vi "main.vi"() -> ()   [LabVIEW 2016]
uses:
  Program Files (x86)/National Instruments/LabVIEW 2016/examples/Instrument IO/Serial/support/Serial - Settings.ctl
  2017-7-21/control1.ctl
  <vilib>/myRIO/Common/Instrument Driver Framework/myRIO v1.0/Encoder/typedefs/Encoder Signal Mode.ctl
  <vilib>/myRIO/Instrument Drivers/Onboard IO/DIO/typedefs/DIO Reference.ctl
  <vilib>/myRIO/Common/Instrument Driver Framework/Utilities/typedefs/myRIO Generic Hardware Reference.ctl
  <vilib>/myRIO/Common/Instrument Driver Framework/Utilities/typedefs/Hardware Version Enum.ctl
  <vilib>/myRIO/Common/Instrument Driver Framework/Utilities/typedefs/myRIO v1.0 Reference.ctl
  <vilib>/myRIO/Common/Instrument Driver Framework/Utilities/typedefs/Generic FPGA Reference.ctl
  <vilib>/myRIO/Common/Instrument Driver Framework/myRIO v1.0/DIO/typedefs/DIO Channels List.ctl
  <vilib>/myRIO/Common/Instrument Driver Framework/myRIO v1.0/DIO/typedefs/DIO Channels Enum.ctl
  <vilib>/userdefined/High Color/nirio_resource_hc.ctl
  <vilib>/myRIO/Common/Instrument Driver Framework/Utilities/vis/Is FPGA Ref Available.vi
  <vilib>/myRIO/Common/Instrument Driver Framework/myRIO v1.0/DIO/vis/myRIO v1.1 Open DIO.vi
  <vilib>/myRIO/Common/Instrument Driver Framework/Utilities/vis/Validate Channels.vi
  <vilib>/myRIO/Common/Instrument Driver Framework/myRIO v1.0/DIO/vis/myRIO v1.0 Reserve DIO.vi
  <vilib>/myRIO/Common/Instrument Driver Framework/myRIO v1.0/Resource Manager/vis/myRIO v1.0 Reserve Channel List.vi
  <vilib>/myRIO/Common/Instrument Driver Framework/myRIO v1.0/DIO/vis/myRIO v1.0 Build MUX Configuration DIO.vi
  <vilib>/myRIO/Common/Instrument Driver Framework/myRIO v1.0/Resource Manager/vis/myRIO v1.0 Reserve Channel.vi
  <vilib>/myRIO/Common/Instrument Driver Framework/myRIO v1.0/Resource Manager/vis/myRIO v1.0 Unreserve Channel.vi
  <vilib>/myRIO/Common/Instrument Driver Framework/myRIO v1.0/Resource Manager/vis/myRIO v1.0 Create Configuration List.vi
  <vilib>/myRIO/Common/Instrument Driver Framework/myRIO v1.0/Resource Manager/vis/myRIO v1.0 Build Mutex Name.vi
  <vilib>/Instr/_visa.llb/VISA Configure Serial Port (Instr).vi
  <vilib>/Utility/error.llb/Error Cluster From Error Code.vi
  <vilib>/myRIO/Common/Instrument Driver Framework/myRIO v1.0/DIO/vis/myRIO v1.0 Write DIO.vi
  <vilib>/myRIO/Common/Instrument Driver Framework/myRIO v1.0/Encoder/vis/myRIO v1.0 Read Encoder.vi
  <vilib>/Utility/VariantDataType/GetNumericInfo.vi
  <vilib>/myRIO/Common/Instrument Driver Framework/myRIO v1.0/myRIO v1.1 Open.vi
  <vilib>/myRIO/Common/Instrument Driver Framework/Utilities/vis/IO Manager.vi
  <vilib>/myRIO/Common/Instrument Driver Framework/Utilities/vis/Configuration Manager.vi
  <vilib>/myRIO/Common/Instrument Driver Framework/myRIO v1.0/Resource Manager/vis/myRIO v1.0 Configure IO.vi
  <vilib>/myRIO/Common/Instrument Driver Framework/myRIO v1.0/myRIO v1.0 Close.vi
  <vilib>/myRIO/Express VI/Onboard IO/DO/DO Express VI.xnode
  <vilib>/myRIO/Instrument Drivers/Onboard IO/DIO/vis/myRIO DIO Open.xnode
  <vilib>/myRIO/Instrument Drivers/Onboard IO/DIO/DIO.lvlib
  <vilib>/myRIO/Instrument Drivers/Onboard IO/Encoder/Encoder.lvlib
panel:
  out "调整的角度1":dbl
  out "长度":i32
  out "4（找球、捡球）":bool
  out "3（移动）":bool
  out "2（投球）":bool
  out "1（捡球）":bool
  out "0（无命令）":bool
  out "收到X坐标":i32
  out "收到Y坐标":i32
  out "收到的角度":dbl
  out "收到的状态":i32
  out "x轴":dbl
  out "Y轴":dbl
  out "Counter Value":i32
  out "x*y":dbl
  out "read buffer":string
  out "读取缓冲区":string
  in  "停止":bool
  in  "写入":bool
  out "角度":dbl
  out "角度 弧度":dbl
  in  "调整":dbl
  out "调整后 角度值":dbl
  in  "A/DIO0 (Pin 11)":bool
  out "建立通信":errorcluster caption="错误输出"
  out "收到的数据":string
  out "发送":string
  out "发送的标志位":string="0"
  out "发送的角度":string
  out "Y轴字符串":string
  out "X轴字符串":string
  # "东南大学篮球机器机器人下位机"
  # "室内定位"
  # "通信"
  # "数据解析"
  # "电子罗盘"
  # "脚轮"
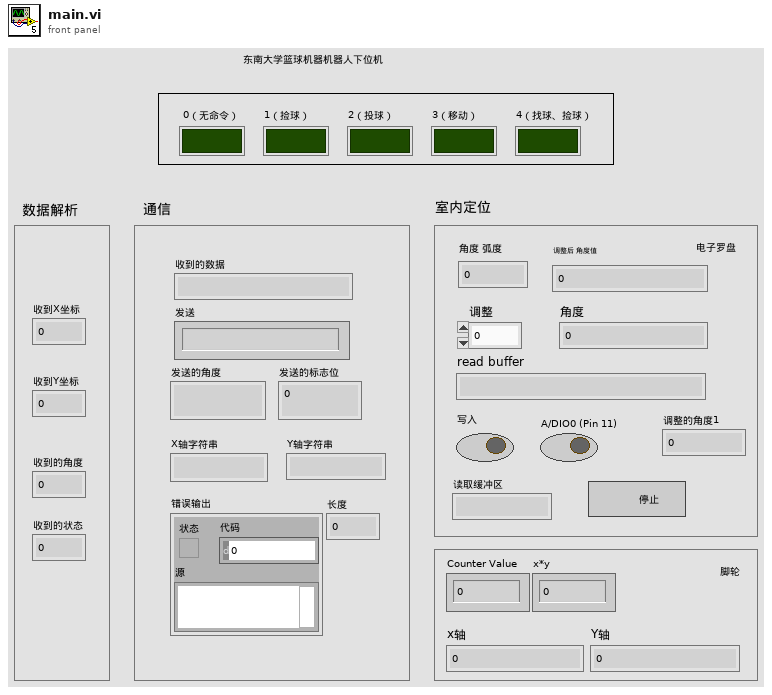
[diagram p1: front panel]
types:
  T1 = typedef "control1.ctl" = cluster{"XON":enum16{"NUL", "SOH", "STX", "ETX", "EOT", "ENQ", "ACK", "BEL", "BS", "HT", "LF", "VT", "FF", "CR", "SO", "SI", "DLE", "DC1", "DC2", "DC3", "DC4", "NAK", "SYN", "ETB", "CAN", "EM", "SUB", "ESC", "FS", "GS", "RS", "US", "SP", "!", "\"", "#", "$", "%", "&", "'", "(", ")", "*", "+", ",", "- (-)", ".", "/", "0", "1", "2", "3", "4", "5", "6", "7", "8", "9", ":", ";", "<", "=", ">", "?", "@", "A", "B", "C", "D", "E", "F", "G", "H", "I", "J", "K", "L", "M", "N", "O", "P", "Q", "R", "S", "T", "U", "V", "W", "X", "Y", "Z", "[", "\\", "]", "^", "_", "`", "a", "b", "c", "d", "e", "f", "g", "h", "i", "j", "k", "l", "m", "n", "o", "p", "q", "r", "s", "t", "u", "v", "w", "x", "y", "z", "{", "|", "}", "~"}, "XOFF":enum16{"NUL", "SOH", "STX", "ETX", "EOT", "ENQ", "ACK", "BEL", "BS", "HT", "LF", "VT", "FF", "CR", "SO", "SI", "DLE", "DC1", "DC2", "DC3", "DC4", "NAK", "SYN", "ETB", "CAN", "EM", "SUB", "ESC", "FS", "GS", "RS", "US", "SP", "!", "\"", "#", "$", "%", "&", "'", "(", ")", "*", "+", ",", "- (-)", ".", "/", "0", "1", "2", "3", "4", "5", "6", "7", "8", "9", ":", ";", "<", "=", ">", "?", "@", "A", "B", "C", "D", "E", "F", "G", "H", "I", "J", "K", "L", "M", "N", "O", "P", "Q", "R", "S", "T", "U", "V", "W", "X", "Y", "Z", "[", "\\", "]", "^", "_", "`", "a", "b", "c", "d", "e", "f", "g", "h", "i", "j", "k", "l", "m", "n", "o", "p", "q", "r", "s", "t", "u", "v", "w", "x", "y", "z", "{", "|", "}", "~"}}
  T2 = typedef "Serial - Settings.ctl" = cluster{"波特率":u32, "数据位":u16, "校验":enum16{"None", "Odd", "Even", "Mark", "Space"}, "停止位":u16, "流控制":u16}
  T3 = typedef "DIO.lvlib/DIO Reference.ctl" = cluster{"myRIO Reference":T4, "DIO Channels List":T8}
  T4 = typedef "myRIO Generic Hardware Reference.ctl" = cluster{"myRIO Model":T5, "myRIO Hardware Reference":T6}
  T5 = typedef "Hardware Version Enum.ctl" = enum16{"Unknown", "myRIO-1900", "myRIO-1950", "roboRIO", "NI ELVIS RIO CM"}
  T6 = typedef "myRIO v1.0 Reference.ctl" = cluster{"Generic FPGA Reference":T7, "Allow multiple opens":bool}
  T7 = typedef "Generic FPGA Reference.ctl" = refnum<k20>
  T8 = typedef "DIO Channels List.ctl" = T9[]
  T9 = typedef "DIO Channels Enum.ctl" = enum16{"Not Connected", "C/DIO0", "C/DIO1", "C/DIO2", "C/DIO3", "C/DIO4", "C/DIO5", "C/DIO6", "C/DIO7", "A/DIO0", "A/DIO1", "A/DIO2", "A/DIO3", "A/DIO4", "A/DIO5", "A/DIO6", "A/DIO7", "A/DIO8", "A/DIO9", "A/DIO10", "A/DIO11", "A/DIO12", "A/DIO13", "A/DIO14", "A/DIO15", "B/DIO0", "B/DIO1", "B/DIO2", "B/DIO3", "B/DIO4", "B/DIO5", "B/DIO6", "B/DIO7", "B/DIO8", "B/DIO9", "B/DIO10", "B/DIO11", "B/DIO12", "B/DIO13", "B/DIO14", "B/DIO15", "LED0", "LED1", "LED2", "LED3", "Button0", "DIO/DIO0", "DIO/DIO1", "DIO/DIO2", "DIO/DIO3", "DIO/DIO4", "DIO/DIO5", "DIO/DIO6", "DIO/DIO7", "DIO/DIO8", "DIO/DIO9", "SPI/CS0", "SPI/CS1", "SPI/CS2", "SPI/CS3", "LED RADIO (Green)", "LED RADIO (Red)", "LED COMM (Green)", "LED COMM (Red)", "LED MODE (Green)", "LED MODE (Red)"}
  T10 = typedef "nirio_resource_hc.ctl" = tag
  T11 = typedef "Encoder Signal Mode.ctl" = enum16{"Quadrature phase signal", "Step and direction signal"}
  T12 = typedef "PWM.lvlib/PWM Reference.ctl" = cluster{"myRIO Reference":T4, "PWM Channels Enum":T13, "PWM Configuration":T14}
  T13 = typedef "PWM Channels Enum.ctl" = enum16{"Not Connected", "C/PWM0", "C/PWM1", "A/PWM0", "A/PWM1", "A/PWM2", "B/PWM0", "B/PWM1", "B/PWM2", "PWM/PWM0", "PWM/PWM1", "PWM/PWM2", "PWM/PWM3", "PWM/PWM4", "PWM/PWM5", "PWM/PWM6", "PWM/PWM7", "PWM/PWM8", "PWM/PWM9"}
  T14 = typedef "PWM.lvlib/PWM Configuration.ctl" = cluster{"Frequency":dbl, "Duty Cycle":dbl}
  T15 = enum16{"NUL", "SOH", "STX", "ETX", "EOT", "ENQ", "ACK", "BEL", "BS", "HT", "LF", "VT", "FF", "CR", "SO", "SI", "DLE", "DC1", "DC2", "DC3", "DC4", "NAK", "SYN", "ETB", "CAN", "EM", "SUB", "ESC", "FS", "GS", "RS", "US", "SP", "!", "\"", "#", "$", "%", "&", "'", "(", ")", "*", "+", ",", "- (-)", ".", "/", "0", "1", "2", "3", "4", "5", "6", "7", "8", "9", ":", ";", "<", "=", ">", "?", "@", "A", "B", "C", "D", "E", "F", "G", "H", "I", "J", "K", "L", "M", "N", "O", "P", "Q", "R", "S", "T", "U", "V", "W", "X", "Y", "Z", "[", "\\", "]", "^", "_", "`", "a", "b", "c", "d", "e", "f", "g", "h", "i", "j", "k", "l", "m", "n", "o", "p", "q", "r", "s", "t", "u", "v", "w", "x", "y", "z", "{", "|", "}", "~"}
  T16 = typedef "Encoder.lvlib/Encoder Reference.ctl" = cluster{"myRIO Reference":T4, "Encoder Channels Enum":T17}
  T17 = typedef "Encoder Channels Enum.ctl" = enum16{"Not Connected", "C/ENC0", "C/ENC1", "A/ENC", "B/ENC", "DIO/ENC0", "DIO/ENC1", "DIO/ENC2", "DIO/ENC3", "DIO/ENC4"}
  T18 = cluster{"PWM Ref Out":T12, "PWM Ref Out":T12, "PWM Ref Out":T12, "PWM Ref Out":T12, "DIO Ref Out":T3}
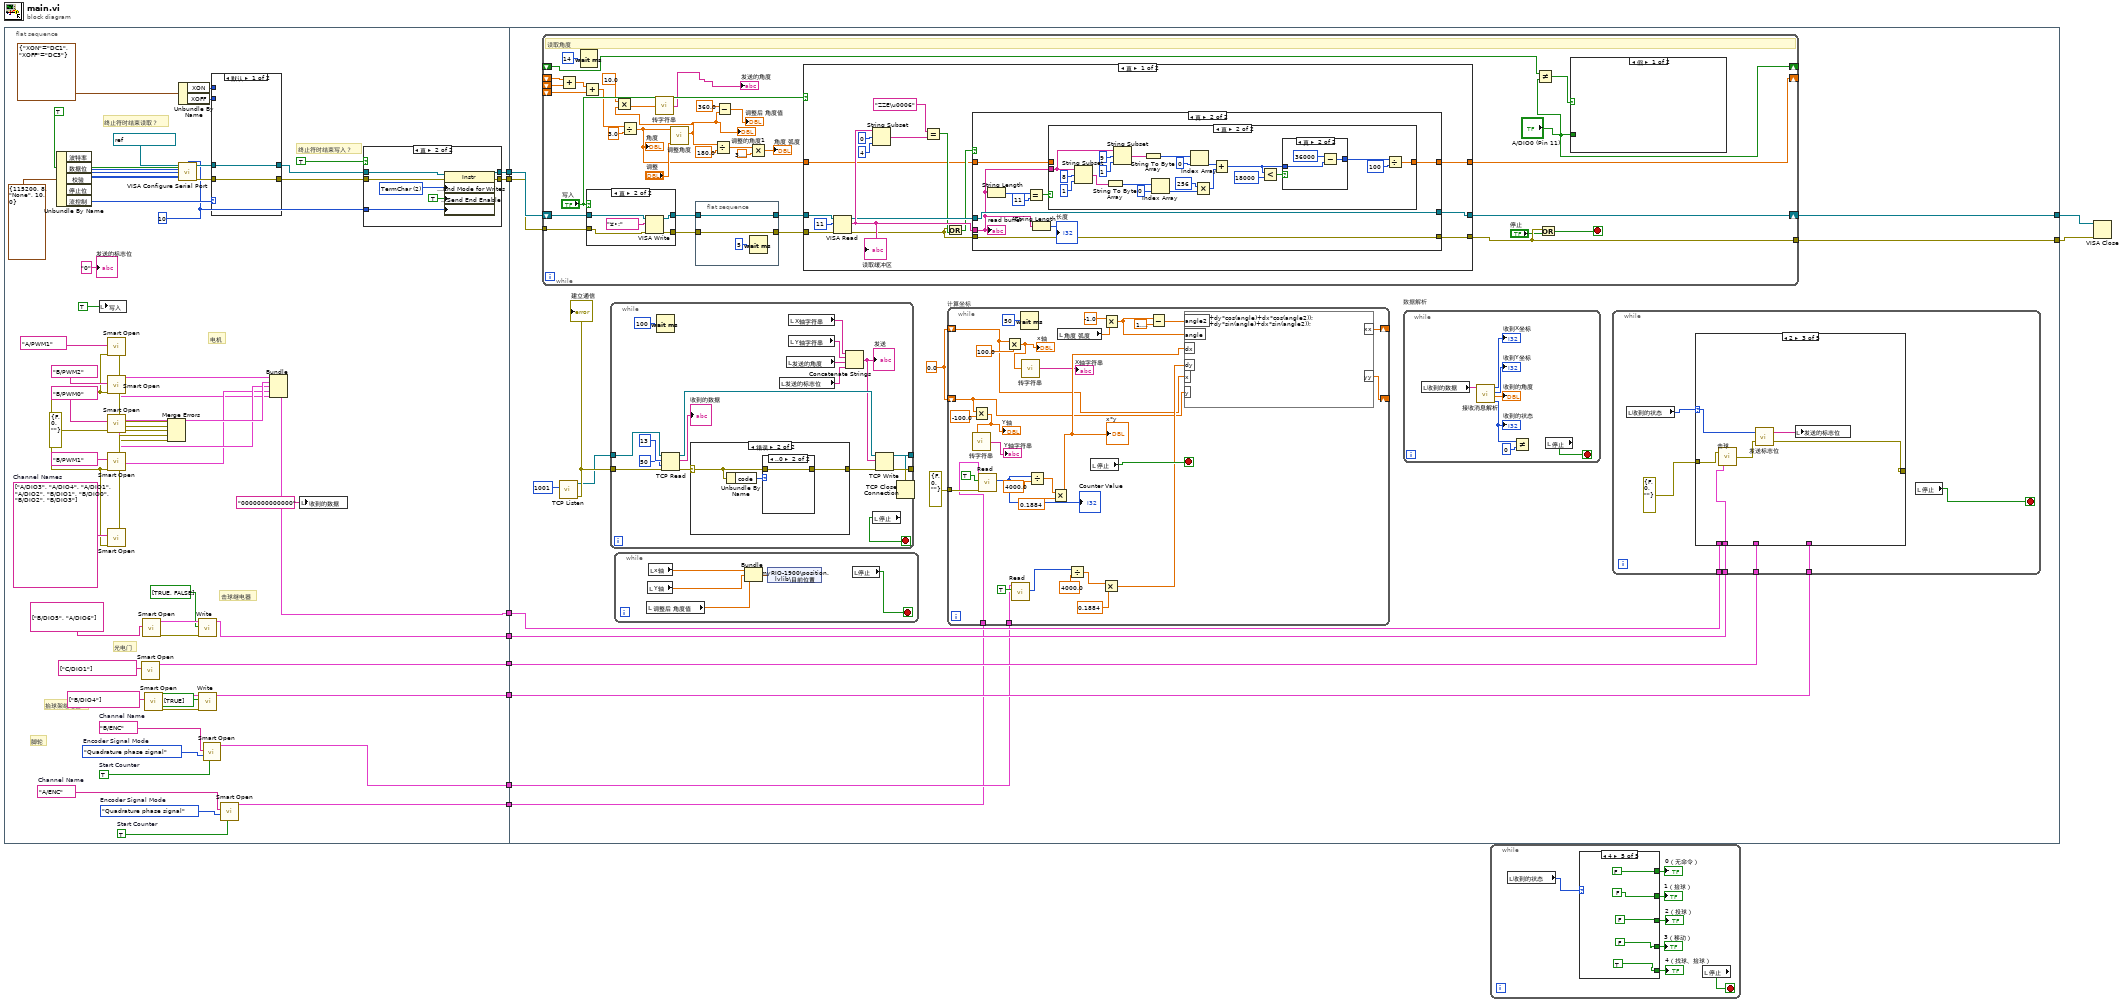
[diagram p0: block diagram]
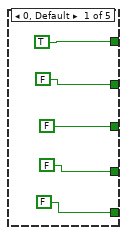
[diagram p2: hidden frame]
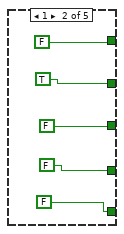
[diagram p3: hidden frame]
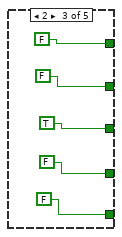
[diagram p4: hidden frame]
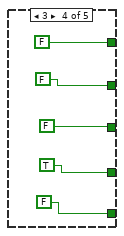
[diagram p5: hidden frame]
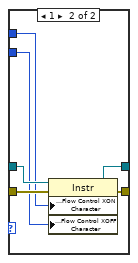
[diagram p7: hidden frame]
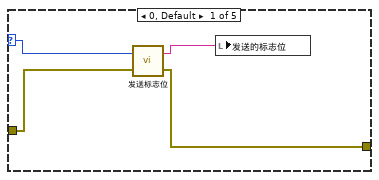
[diagram p8: hidden frame]
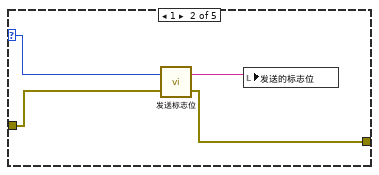
[diagram p9: hidden frame]
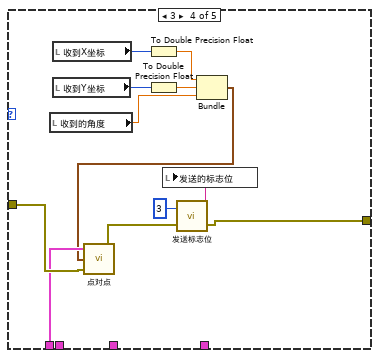
[diagram p10: hidden frame]
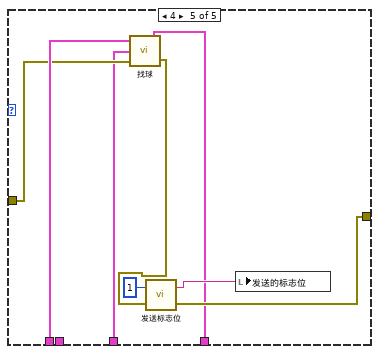
[diagram p11: hidden frame]
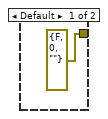
[diagram p13: hidden frame]
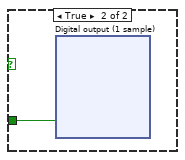
[diagram p14: hidden frame]
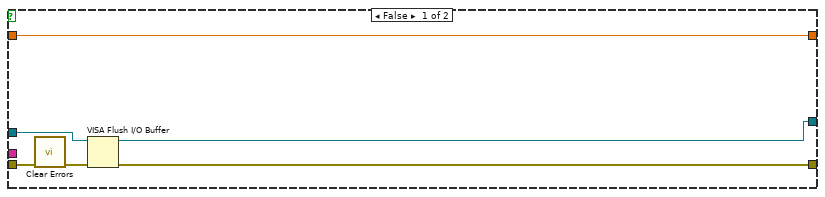
[diagram p16: hidden frame]
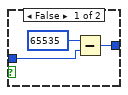
[diagram p18: hidden frame]
diagram:
  n1 = flat-sequence {
    tunnel: [w34] -> w10
    tunnel: [w33] -> w9
    tunnel: [w32] -> w6
    tunnel: [w26] -> w5
    tunnel: [w24] -> w4
    tunnel: [w19] -> w3
    tunnel: [w15] -> w2
    tunnel: [w11] -> w1
    tunnel: w10 -> [w103]
    tunnel: w9 -> [w102]
    tunnel: [w101] -> w8
    tunnel: [w100] -> w7
    tunnel: w6 -> [w92]
    tunnel: w5 -> [w91]
    tunnel: w4 -> [w90]
    tunnel: w3 -> [w89]
    tunnel: w2 -> [w88]
    tunnel: w1 -> [w87]
    frame #0 {
      w12 = TRUE  # Start Counter
      w13 = Encoder_Signal_Mode."Quadrature phase signal"  # Encoder Signal Mode
      w14 = tag "A/ENC"  # Channel Name
      w16 = TRUE  # Start Counter
      w17 = Encoder_Signal_Mode."Quadrature phase signal"  # Encoder Signal Mode
      w18 = tag "B/ENC"  # Channel Name
      w62 = errorcluster {"status"=FALSE, "code"=0, "source"=""} ("错误输入")
      w37 = u8 10 ("终止符")
      w63 = tag[] ["A/DIO3", "A/DIO4", "A/DIO1", "A/DIO2", "B/DIO1", "B/DIO0", "B/DIO2", "B/DIO3"]  # Channel Names
      # "脚轮"
      # "抬球架继电器"
      # "光电门"
      # "电机"
      # "击球继电器"
      # "终止符时结束读取？"
      # "终止符时结束写入？"
      n2 = Unbundle By Name(T2 {"波特率"=115200, "数据位"=8, "校验"=enum."None", "停止位"=10, "流控制"=0} ("串口设置")) -> ("波特率"=w44:u32, "数据位"=w45:u16, "校验"=w46:enum16{"None", "Odd", "Even", "Mark", "Space"}, "停止位"=w47:u16, "流控制"=w42:u16)
      n3 = local write "写入"(TRUE ("写入")) -> ()
      n4 = call <vilib>:"Smart Open.vi"("error in (no error)"=w62, "Channel Name"=tag "A/PWM1") -> ("error out"=w61:errorcluster, "PWM Ref Out"=w56:T12)  [unwired: 8 in]
      n5 = call <vilib>:"Smart Open.vi"("error in (no error)"=w62, "Channel Name"=tag "B/PWM2") -> ("error out"=w60:errorcluster, "PWM Ref Out"=w55:T12)  [unwired: 8 in]
      n6 = call <vilib>:"Smart Open.vi"("error in (no error)"=w62, "Channel Name"=tag "B/PWM0") -> ("error out"=w59:errorcluster, "PWM Ref Out"=w54:T12)  [unwired: 8 in]
      n7 = call <vilib>:"Smart Open.vi"("error in (no error)"=w62, "Channel Name"=tag "B/PWM1") -> ("error out"=w58:errorcluster, "PWM Ref Out"=w53:T12)  [unwired: 8 in]
      n8 = call <vilib>:"Smart Open.vi"("error in (no error)"=w62, "Channel Names"=w63) -> ("error out"=w57:errorcluster, "DIO Ref Out"=w52:T3)  [unwired: 8 in]
      n9 = call <vilib>:"Smart Open.vi"("Channel Names"=tag[] ["C/DIO1"]) -> ("DIO Ref Out"=w24:T3)  [unwired: 9 in, 1 out]
      n10 = call <vilib>:"Smart Open.vi"("Channel Names"=tag[] ["B/DIO5", "A/DIO6"]) -> ("error out"=w27:errorcluster, "DIO Ref Out"=w29:T3)  [unwired: 9 in]
      n11 = call <vilib>:"Smart Open.vi"("Channel Names"=tag[] ["B/DIO4"]) -> ("error out"=w21:errorcluster, "DIO Ref Out"=w22:T3)  [unwired: 9 in]
      n12 = Merge Errors(w61, w60, w59, w58, w57) -> ()  [unwired: 1 out]
      n13 = Unbundle By Name(T1 {"XON"=enum."DC1", "XOFF"=enum."DC3"}) -> ("XON"=w41:T15, "XOFF"=w40:T15)
      n14 = call-poly "VISA Configure Serial Port"("VISA resource name"=refnum<visa-resource-name> "ASRL2::INSTR" ("VISA资源名称"), "termination char\n(0xA = '\\n' = LF)"=w37, "Enable Termination\nChar (T)"=TRUE, "baud rate (9600)"=w44, "data bits (8)"=w45, "parity (0:none)"=w46, "stop bits (10: 1 bit)"=w47, "flow control (0:none)"=w42) -> ("VISA resource name out"=w48:refnum<visa-resource-name>, "error out"=w49:errorcluster)  [unwired: 2 in, 4 out]
      n15 = call <vilib>:"Write.vi"("error in (no error)"=w27, "Values"=bool[] [TRUE, FALSE], "DIO Ref In"=w29) -> ("DIO Ref Out"=w26:T3)  [unwired: 6 in, 1 out]
      n16 = call <vilib>:"Write.vi"("error in (no error)"=w21, "Values"=bool[] [TRUE], "DIO Ref In"=w22) -> ("DIO Ref Out"=w19:T3)  [unwired: 6 in, 1 out]
      n17 = call <vilib>:"Smart Open.vi"("Start Counter"=w16, "Encoder Signal Mode"=w17, "Channel Name"=w18) -> ("Encoder Ref Out"=w15:T16)  [unwired: 7 in, 1 out]
      n18 = case shown="默认" w42 {
        tunnel: [w79 w86] -> w39
        tunnel: [w80 w85] -> w38
        tunnel: w49 -> [w79 w84]
        tunnel: w48 -> [w80 w83]
        tunnel: w41 -> [_ w82]
        tunnel: w40 -> [_ w81]
        frame Default {
        }
        frame 1 {
          n19 = property class="Instr"(reference=w83, error in=w84, "Serial Settings:Flow Control XON Character"=w82, "Serial Settings:Flow Control XOFF Character"=w81) -> (reference out=w85:refnum<visa-resource-name>, error out=w86:errorcluster)
        }
      }
      n20 = call <vilib>:"Smart Open.vi"("Start Counter"=w12, "Encoder Signal Mode"=w13, "Channel Name"=w14) -> ("Encoder Ref Out"=w11:T16)  [unwired: 7 in, 1 out]
      n21 = Bundle("PWM Ref Out"=w56, "PWM Ref Out"=w55, "PWM Ref Out"=w54, "PWM Ref Out"=w53, "DIO Ref Out"=w52) -> (w32:T18)  [unwired: 1 in]
      n22 = local write "收到的数据"("0000000000000" ("收到的数据")) -> ()
      n23 = case shown="真" TRUE {
        tunnel: w38 -> [w70 w78]
        tunnel: w39 -> [w71 w77]
        tunnel: [w70 w76] -> w34
        tunnel: [w71 w75] -> w33
        tunnel: w37 -> [_ w73]
        frame False {
        }
        frame True {
          w74 = u16 2 items=["None", "LastBit", "TermChar", "Break"] ("Serial Settings:Serial End Mode for Writes")
          n24 = property class="Instr"(reference=w78, error in=w77, "Serial Settings:End Mode for Writes"=w74, "Message Based Settings:Send End Enable"=TRUE, "Message Based Settings:Termination Character"=w73) -> (reference out=w76:refnum<visa-resource-name>, error out=w75:errorcluster)
        }
      }
      "发送的标志位" <- "0" ("发送的标志位")
    }
    frame #1 {
      w94 = 0.0
      n25 = while {
        shift-right: [w245] -> w100
        shift-left: w103 -> [w244]
        tunnel: [w242] -> w101
        shift-right: [w234] -> _
        shift-left: _ -> [w233]
        shift-left: _ -> [w232]
        shift-left: _ -> [w230]
        shift-right: ["A/DIO0 (Pin 11)"] -> _
        shift-left: _ -> [w220]
        tunnel: w102 -> [w219]
        stop <- w243 stop-if-true
        # "读取角度"
        n26 = Add(x=w233, y=w232) -> (x+y=w231:dbl)
        n27 = Wait (ms)(milliseconds to wait=u32 14) -> ()  [unwired: 1 out]
        n28 = Add(x=w231, y=w230) -> (x+y=w229:dbl)
        n29 = case shown="真" "写入" {
          tunnel: w244 -> [w286 w290]
          tunnel: [w286 w289] -> w240
          tunnel: [w285 w288] -> w239
          tunnel: w219 -> [w285 w287]
          frame False {
          }
          frame True {
            n30 = VISA Write(VISA resource name=w290, write buffer="¥•:" ("命令"), error in (no error)=w287) -> (VISA resource name out=w289:refnum<visa-resource-name>, error out=w288:errorcluster)  [unwired: 1 out]
          }
        }
        n31 = Divide(x=w229, y=3.0) -> (x/y=w215:dbl)
        "角度" <- w215
        n32 = call "调整角度.vi"("调整"="调整", "原角度"=w215) -> ("调整后 角度值"=w212:dbl)  [unwired: 9 in]
        "调整的角度1" <- w212
        n33 = Multiply(x=10.0, y=w212) -> (x*y=w217:dbl)
        n34 = call "转字符串.vi"("输入"=w217) -> ("结果字符串"=→"发送的角度":string)
        n35 = flat-sequence {
          tunnel: w240 -> [w283]
          tunnel: w239 -> [w284]
          tunnel: [w284] -> w238
          tunnel: [w283] -> w237
          frame #0 {
            n36 = Wait (ms)(milliseconds to wait=u32 5) -> ()  [unwired: 1 out]
          }
        }
        n37 = Divide(x=w212, y=180.0) -> (x/y=w225:dbl)
        n38 = Subtract(x=360.0, y=w212) -> (x-y=→"调整后 角度值":dbl)
        n39 = Multiply(x=w225, y=3.141592653589793) -> (x*y=→"角度 弧度":dbl)
        n40 = case shown="真" "写入" {
          tunnel: [w300 w352] -> w245
          tunnel: [w294 w353] -> w242
          tunnel: w238 -> [w299 w353]
          tunnel: w237 -> [w298 w352]
          tunnel: [w293 w351] -> w234
          tunnel: w215 -> [w292 w351]
          frame True {
            n41 = VISA Read(VISA resource name=w298, byte count=u32 11 ("读数"), error in (no error)=w299) -> (VISA resource name out=w301:refnum<visa-resource-name>, read buffer=w302:string, error out=w295:errorcluster)  [unwired: 1 out]
            "读取缓冲区" <- w302
            n42 = String Subset(string=w302, offset (0)=0 ("偏移量(0)"), length (rest)=4 ("长度（剩余）")) -> (substring=w304:string)
            n43 = Equal?(x="ZZE\u0006", y=w304) -> (x = y?=w297:bool)
            n44 = Or(x=w295, y=w297) -> (x .or. y?=w296:bool)
            n45 = case shown="真" w296 {
              tunnel: w302 -> [_ w315]
              tunnel: w301 -> [w313 w322]
              tunnel: [w312 w322] -> w300
              tunnel: w295 -> [w311 w321]
              tunnel: [w309 w321] -> w294
              tunnel: [w308 w317] -> w293
              tunnel: w292 -> [w308 w316]
              frame False {
                n46 = call <vilib>:"Clear Errors.vi"("error in (no error)"=w311) -> ("error out"=w310:errorcluster)  [unwired: 5 in, 1 out]
                n47 = VISA Flush I/O Buffer(VISA resource name=w313, error in (no error)=w310) -> (VISA resource name out=w312:refnum<visa-resource-name>, error out=w309:errorcluster)  [unwired: 1 in]
              }
              frame True {
                n48 = String Length(string=w315) -> (length=w318:i32)
                n49 = Equal?(x=w318, y=11) -> (x = y?=w320:bool)
                n50 = String Length(string=w315) -> (length=→"长度":i32)
                n51 = case shown="真" w320 {
                  tunnel: w315 -> [_ w332]
                  tunnel: [w323 w324] -> w317
                  tunnel: w316 -> [w323 _]
                  frame False {
                  }
                  frame True {
                    n52 = String Subset(string=w332, offset (0)=8 ("偏移量(0)"), length (rest)=1 ("长度（剩余）")) -> (substring=w342:string)
                    n53 = String To Byte Array(string=w342) -> (unsigned byte array=w341:u8[])
                    n54 = String Subset(string=w332, offset (0)=9 ("偏移量(0)"), length (rest)=1 ("长度（剩余）")) -> (substring=w335:string)
                    n55 = String To Byte Array(string=w335) -> (unsigned byte array=w336:u8[])
                    n56 = Index Array(array=w341, index=0 ("索引")) -> (element=w339:u8)
                    n57 = Index Array(array=w336, index=0 ("索引")) -> (element=w331:u8)
                    n58 = Multiply(x=256, y=w339) -> (x*y=w330:i32)
                    n59 = Add(x=w331, y=w330) -> (x+y=w327:i32)
                    n60 = Less?(x=w327, y=18000) -> (x < y?=w328:bool)
                    n61 = case shown="真" w328 {
                      tunnel: w327 -> [w345 w350]
                      tunnel: [w347 w348] -> w326
                      frame False {
                        n62 = Subtract(x=65535 ("y"), y=w345) -> (x-y=w347:i32)
                      }
                      frame True {
                        n63 = Subtract(x=36000, y=w350) -> (x-y=w348:i32)
                      }
                    }
                    n64 = Divide(x=w326, y=100) -> (x/y=w324:dbl)
                  }
                }
                "read buffer" <- w315
              }
            }
          }
          frame False {
          }
        }
        n65 = Not Equal?(x=w220, y="A/DIO0 (Pin 11)") -> (x != y?=w222:bool)
        n66 = Or(x=w242, y="停止") -> (x .or. y?=w243:bool)
        n67 = case shown="假" w222 {
          tunnel: "A/DIO0 (Pin 11)" -> [_ w246]
          frame False {
          }
          frame True {
            n68 = xnode "Digital output (1 sample)"("A/DIO1 (Pin 13)"=w246) -> ()  [unwired: 1 in, 1 out]
          }
        }
      }
      n69 = call <vilib>:"TCP Listen.vi"("port"=u16 1001 ("远程端口或服务名称")) -> ("error out"=w99:errorcluster, "connection ID"=w95:refnum<k5>)  [unwired: 6 in, 3 out]
      "建立通信" <- w99
      n70 = while {
        tunnel: w95 -> [w205]
        tunnel: w99 -> [w204]
        tunnel: [w199] -> w96
        tunnel: [w197] -> w97
        stop <- w189 stop-if-true
        n71 = Wait (ms)(milliseconds to wait=100) -> ()  [unwired: 1 out]
        n72 = TCP Read(connection ID=w205, bytes to read=13 ("读取的字节"), error in (no error)=w204, 9:50) -> (connection ID out=w200:refnum<k5>, data out=→"收到的数据":string, error out=w202:errorcluster)  [unwired: 1 in]
        n73 = case shown="错误" w202 {
          selector: w202 -> [w206 w207]
          tunnel: [w206 w208] -> w198
          frame No Error {
          }
          frame Error {
            n74 = Unbundle By Name(w207) -> ("code"=w209:i32)
            n75 = case shown="..0" w209 {
              tunnel: [errorcluster {"status"=FALSE, "code"=0, "source"=""} ("error IO") w211] -> w208
              tunnel: w207 -> [_ w211]
              frame Default {
              }
              frame ..0 {
              }
            }
          }
        }
        n76 = local read "发送的标志位"() -> (w191:string)
        n77 = local read "发送的角度"() -> (w190:string)
        n78 = local read "X轴字符串"() -> (w194:string)
        n79 = local read "Y轴字符串"() -> (w193:string)
        n80 = Concatenate Strings(w194, w193, w190, w191) -> (w192:string)
        "发送" <- w192
        n81 = local read "停止"() -> (w189:bool)
        n82 = TCP Write(connection ID=w200, data in=w192, error in (no error)=w198) -> (connection ID out=w199:refnum<k5>, error out=w197:errorcluster)  [unwired: 1 in, 1 out]
      }
      n83 = while {
        stop <- w104 stop-if-true
        n84 = local read "调整后 角度值"() -> (w106:dbl)
        n85 = local read "Y轴"() -> (w107:dbl)
        n86 = local read "x轴"() -> (w108:dbl)
        n87 = Bundle("x轴"=w108, "Y轴"=w107, "调整后 角度值"=w106) -> (w105:cluster{"x轴":dbl, "Y轴":dbl, "调整后 角度值":dbl})  [unwired: 1 in]
        n88 = shared-variable "myRIO-1900\\position.lvlib\\目前位置"(w105) -> ()  [unwired: 1 in, 1 out]
        n89 = local read "停止"() -> (w104:bool)
      }
      n90 = TCP Close Connection(connection ID=w96, error in (no error)=w97) -> ()  [unwired: 1 in, 2 out]
      n91 = while "计算坐标" {
        shift-right: [w187] -> _
        shift-left: w94 -> [w171]
        shift-right: [w186] -> _
        shift-left: w94 -> [w172]
        tunnel: errorcluster {"status"=FALSE, "code"=0, "source"=""} ("错误常量") -> [w161]
        tunnel: w88 -> [w163]
        tunnel: w87 -> [w159]
        stop <- w188 stop-if-true
        n92 = Multiply(x=w172, y=-100.0) -> (x*y=w158:dbl)
        "Y轴" <- w158
        n93 = call "转字符串.vi"("输入"=w158) -> ("结果字符串"=→"Y轴字符串":string)
        n94 = call <vilib>:"Read.vi"("error in (no error)"=w161, "Reset Counter"=TRUE, "Encoder Ref In"=w159) -> ("Counter Value"=w162:i32)  [unwired: 4 in, 4 out]
        "Counter Value" <- w162
        n95 = Multiply(x=w171, y=100.0) -> (x*y=w157:dbl)
        "x轴" <- w157
        n96 = call <vilib>:"Read.vi"("Reset Counter"=TRUE, "Encoder Ref In"=w163) -> ("Counter Value"=w164:i32)  [unwired: 5 in, 4 out]
        n97 = Wait (ms)(milliseconds to wait=u32 50 ("等待时间（毫秒）")) -> ()  [unwired: 1 out]
        n98 = call "转字符串.vi"("输入"=w157) -> ("结果字符串"=→"X轴字符串":string)
        n99 = Divide(x=w162, y=4000.0) -> (x/y=w182:dbl)
        n100 = Multiply(x=w182, y=0.1884) -> (x*y=w180:dbl)
        "x*y" <- w180
        n101 = local read "角度 弧度"() -> (w170:dbl)
        n102 = Divide(x=w164, y=4000.0) -> (x/y=w178:dbl)
        n103 = local read "停止"() -> (w188:bool)
        n104 = Multiply(x=w178, y=0.1884) -> (x*y=w176:dbl)
        n105 = Multiply(x=-1.0, y=w170) -> (x*y=w168:dbl)
        n106 = Subtract(x=w168, y=1.5707963267948966) -> (x-y=w185:dbl)
        n107 = formula code="xx=(x+dy*cos(angle)+dx*cos(angle2));\nyy=(y+dy*sin(angle)+dx*sin(angle2));"("angle"=w168, "dx"=w180, "dy"=w176, "x"=w171, "y"=w172, "angle2"=w185) -> ("xx"=w187:dbl, "yy"=w186:dbl)
      }
      n108 = while "数据解析" {
        stop <- w156 stop-if-true
        n109 = local read "收到的数据"() -> (w150:string)
        n110 = call "接收消息解析.vi"("上位机消息"=w150) -> ("状态"=w155:i32, "角度"=→"收到的角度":dbl, "Y"=→"收到Y坐标":i32, "X"=→"收到X坐标":i32)  [unwired: 7 in]
        "收到的状态" <- w155
        n111 = Not Equal?(x=w155, y=0) -> ()  [unwired: 1 out]
        n112 = local read "停止"() -> (w156:bool)
      }
      n113 = while {
        tunnel: w92 -> [w112]
        tunnel: w91 -> [w111]
        tunnel: w90 -> [w110]
        tunnel: w89 -> [w109]
        stop <- w115 stop-if-true
        n114 = local read "收到的状态"() -> (w113:i32)
        n115 = case shown="2" w113 {
          selector: w113 -> [w119 w123 w127 _ _]
          tunnel: errorcluster {"status"=FALSE, "code"=0, "source"=""} ("error out") -> [w117 w121 w125 w139 w144]
          tunnel: [w116 w120 w128 w130 w148] -> _
          tunnel: w112 -> [_ _ _ w137 w145]
          tunnel: w111 -> [_ _ w124 _ _]
          tunnel: w110 -> [_ _ _ _ w143]
          tunnel: w109 -> [_ _ _ _ w142]
          frame 0, Default {
            n116 = call "发送标志位.vi"("error out 2"=w117, "数值"=w119) -> ("error out"=w116:errorcluster, "十进制整型字符串"=w118:string)
            n117 = local write "发送的标志位"(w118) -> ()
          }
          frame 1 {
            n118 = call "发送标志位.vi"("error out 2"=w121, "数值"=w123) -> ("error out"=w120:errorcluster, "十进制整型字符串"=w122:string)
            n119 = local write "发送的标志位"(w122) -> ()
          }
          frame 2 {
            n120 = call "击球.vi"("DIO Ref Out"=w124, "error in (no error)"=w125) -> ("error out"=w126:errorcluster)
            n121 = call "发送标志位.vi"("error out 2"=w126, "数值"=w127) -> ("error out"=w128:errorcluster, "十进制整型字符串"=w129:string)
            n122 = local write "发送的标志位"(w129) -> ()
          }
          frame 3 {
            n123 = local read "收到的角度"() -> (w132:dbl)
            n124 = local read "收到X坐标"() -> (w136:i32)
            n125 = local read "收到Y坐标"() -> (w135:i32)
            n126 = To Double Precision Float(number=w136) -> (double precision float=w134:dbl)
            n127 = To Double Precision Float(number=w135) -> (double precision float=w133:dbl)
            n128 = Bundle(w134, w133, "收到的角度"=w132) -> (w131:cluster{dbl, dbl, "收到的角度":dbl})  [unwired: 1 in]
            n129 = call "点对点.vi"("错误输入"=w139, "目标位置"=w131, "I/O"=w137) -> ("错误输出"=w138:errorcluster)
            n130 = call "发送标志位.vi"("error out 2"=w138, "数值"=3) -> ("error out"=w130:errorcluster, "十进制整型字符串"=w140:string)
            n131 = local write "发送的标志位"(w140) -> ()
          }
          frame 4 {
            n132 = call "找球.vi"("抬球电机继电器"=w142, "错误输入"=w144, "光电门"=w143, "I/O"=w145) -> ("错误输出"=w146:errorcluster)
            n133 = call "发送标志位.vi"("error out 2"=w146, "数值"=1) -> ("error out"=w148:errorcluster, "十进制整型字符串"=w149:string)
            n134 = local write "发送的标志位"(w149) -> ()
          }
        }
        n135 = local read "停止"() -> (w115:bool)
      }
    }
  }
  n136 = while {
    stop <- w359 stop-if-true
    n137 = local read "收到的状态"() -> (w360:i32)
    n138 = case shown="4" w360 {
      tunnel: [TRUE FALSE FALSE FALSE FALSE] -> w358
      tunnel: [FALSE TRUE FALSE FALSE FALSE] -> w357
      tunnel: [FALSE FALSE TRUE FALSE FALSE] -> w356
      tunnel: [FALSE FALSE FALSE TRUE FALSE] -> w355
      tunnel: [FALSE FALSE FALSE FALSE TRUE] -> w354
      frame 0, Default {
      }
      frame 1 {
      }
      frame 2 {
      }
      frame 3 {
      }
      frame 4 {
      }
    }
    "0（无命令）" <- w358
    "1（捡球）" <- w357
    "2（投球）" <- w356
    "3（移动）" <- w355
    "4（找球、捡球）" <- w354
    n139 = local read "停止"() -> (w359:bool)
  }
  n140 = VISA Close(VISA resource name=w7, error in (no error)=w8) -> ()  [unwired: 1 out]
